vi "picoquant_write_external_stop_event.vi"(8 "error in (no error)":errorcluster, 10 "external_stop_event":refnum<event-registration>, 11 "picoquant_generic in":refnum<class "picoquant_generic.lvclass">) -> (0 "error out":errorcluster, 3 "picoquant_generic out":refnum<class "picoquant_generic.lvclass">)   [LabVIEW 2015, in "picoquant_generic.lvclass"]
uses:
  picoquant_generic.lvclass
  picoquant_generic.lvclass/picoquant_generic.ctl
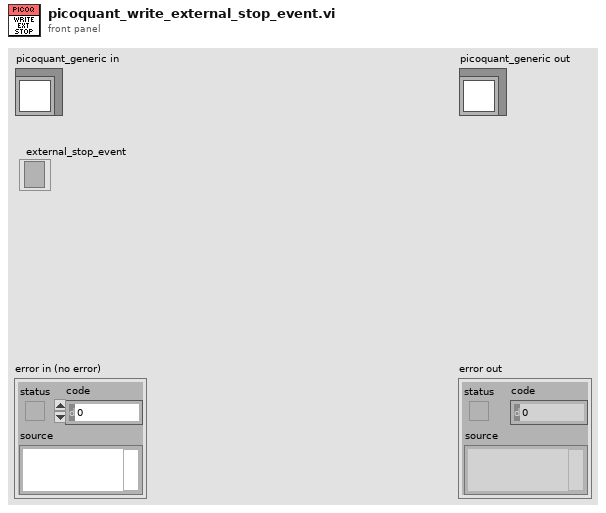
[diagram p1: front panel]
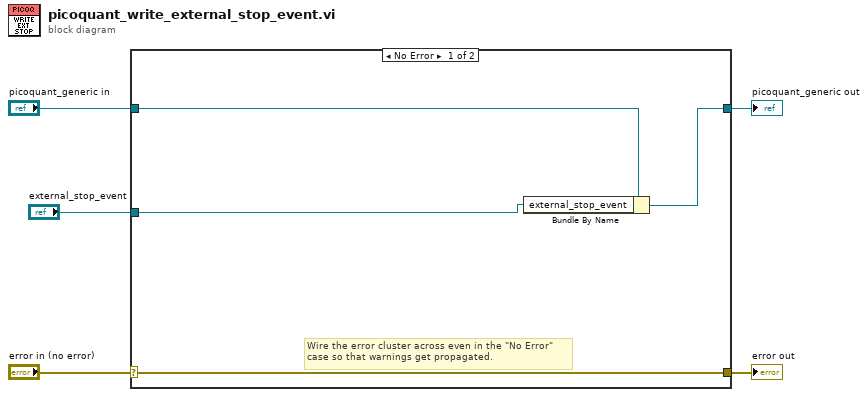
[diagram p0: block diagram]
diagram:
  n1 = case shown="No Error" "error in (no error)" {
    selector: "error in (no error)" -> [w9 w11]
    tunnel: [w9 w11] -> w4
    tunnel: [w6 w10] -> w2
    tunnel: "picoquant_generic in" -> [w7 w10]
    tunnel: "external_stop_event" -> [w8 _]
    frame No Error {
      # "Wire the error cluster across even in the \"No Error\"\ncase so that warnings get propagated."
      n2 = Bundle By Name(cluster=w7, "external_stop_event"=w8) -> (w6:refnum<class "picoquant_generic.lvclass">)
    }
    frame Error {
    }
  }
  "error out" <- w4
  "picoquant_generic out" <- w2
